vi "Menu Response.vi"(8 "error in (no error)":errorcluster, 10 "Menu Tag":string, 11 "Main in":refnum<class "Main.lvclass">) -> (0 "error out":errorcluster, 3 "Main out":refnum<class "Main.lvclass">)   [LabVIEW 2023, in "Main.lvlib" / "Main.lvclass"]
uses:
  Library/Main.lvclass
  Main Messages/Toggle Component Display Msg/Toggle Component Display Msg.lvclass/Toggle Component Display Msg.ctl
  builds/Framework/Engine.lvlibp/Engine/Accessors/Read Self Q.vi
  Custom Controls/Components.vi
  builds/Framework/Actor Framework.lvlibp/1abvi3w/vi.lib/ActorFramework/Message Enqueuer/Enqueue.vi
  builds/Framework/Actor Framework.lvlibp/1abvi3w/vi.lib/ActorFramework/Message Enqueuer/Message Enqueuer.lvclass
  <vilib>/ErrorRing/Error Ring.xnode
  Main Messages/Toggle Component Display Msg/Toggle Component Display Msg.lvclass
  Library/Main.lvclass/Main.ctl
  builds/Framework/Engine.lvlibp/Engine/Library/Engine.lvclass
  builds/Framework/Actor Framework.lvlibp/1abvi3w/vi.lib/ActorFramework/Stop Msg/Stop Msg.lvclass
  C:/Users/Public/Documents/Development/builds/Framework/Engine.lvlibp/Managed Actor/Library/Managed Actor.lvclass
  C:/Users/Public/Documents/Development/builds/Framework/Engine.lvlibp/Engine/Library/Engine.lvclass
  C:/Users/Public/Documents/Development/builds/Framework/Panel Manager.lvlibp/Library/Panel Actor.lvclass
  C:/Users/Public/Documents/Development/builds/Framework/Monitored Actor.lvlibp/Actor Monitor/Actor Monitor/Actor Monitor.lvclass
  C:/Users/Public/Documents/Development/builds/Framework/Actor Framework.lvlibp/1abvi3w/vi.lib/ActorFramework/Actor/Actor.lvclass
  C:/Users/Public/Documents/Development/Application/Main/Library/Main.lvclass
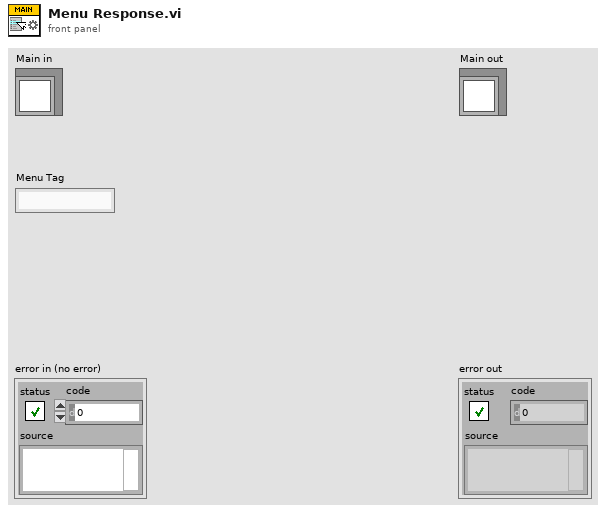
[diagram p1: front panel]
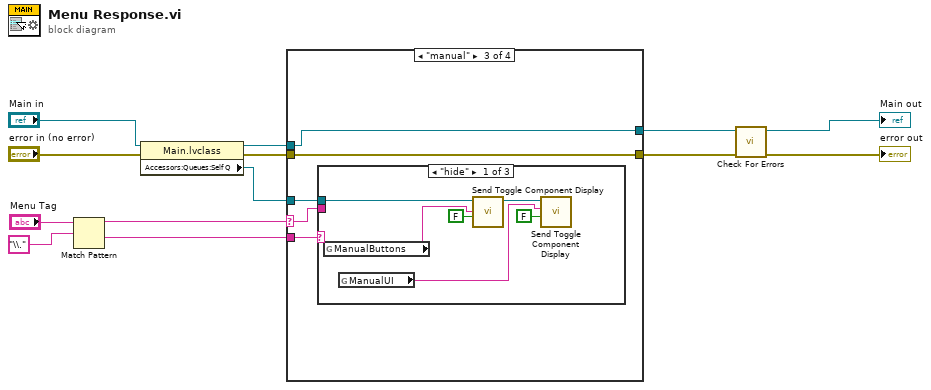
[diagram p0: block diagram]
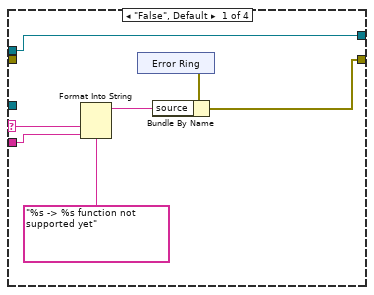
[diagram p2: hidden frame]
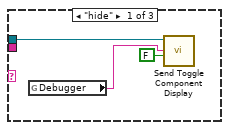
[diagram p4: hidden frame]
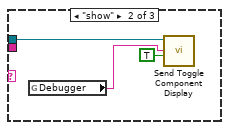
[diagram p5: hidden frame]
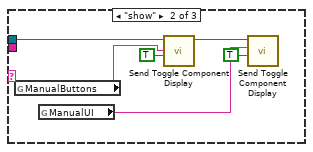
[diagram p6: hidden frame]
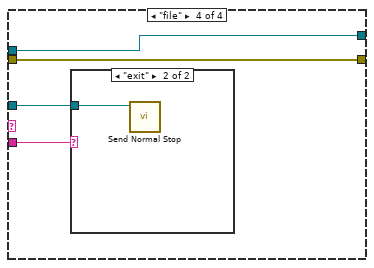
[diagram p8: hidden frame]
diagram:
  n1 = Match Pattern(string="Menu Tag", regular expression="\\.") -> (before substring=w10:string, after substring=w1:string)  [unwired: 1 in, 2 out]
  n2 = property class="Main.lvclass"(reference="Main in", error in="error in (no error)") -> (reference out=w9:refnum<class "Main.lvclass">, error out=w8:errorcluster, "Accessors:Queues:Self Q"=w2:refnum<class "Message Enqueuer.lvclass">)
  n3 = case shown="\"manual\"" w10 {
    selector: w10 -> [w15 w22 w33 _]
    tunnel: w9 -> [w20 w24 w35 w53]
    tunnel: w8 -> [_ w23 w34 w52]
    tunnel: [w20 w24 w35 w53] -> w5
    tunnel: [w16 w23 w34 w52] -> w4
    tunnel: w2 -> [_ w25 w36 w50]
    tunnel: w1 -> [w14 w26 w37 w51]
    frame "False", Default {
      n4 = Format Into String(format string="%s -> %s function not supported yet", w15, w14) -> (resulting string=w17:string)  [unwired: 2 in, 1 out]
      n5 = xnode "Error Ring"() -> ("error out"=w19:errorcluster)
      n6 = Bundle By Name(cluster=w19, "source"=w17) -> (w16:errorcluster)
    }
    frame "debugger" {
      n7 = case shown="Default" w26 {
        tunnel: w25 -> [w29 w32 _]
        tunnel: w22 -> [_ _ _]
        frame "hide" {
          n8 = global read "Components.vi" "Debugger"() -> (w27:string)
          n9 = call "Send Toggle Component Display.vi"("Show"=FALSE, "Identifier"=w27, "Message Enqueuer"=w29) -> ()  [unwired: 7 in, 2 out]
        }
        frame "show" {
          n10 = global read "Components.vi" "Debugger"() -> (w30:string)
          n11 = call "Send Toggle Component Display.vi"("Show"=TRUE, "Identifier"=w30, "Message Enqueuer"=w32) -> ()  [unwired: 7 in, 2 out]
        }
        frame Default {
        }
      }
    }
    frame "manual" {
      n12 = case shown="\"hide\"" w37 {
        tunnel: w36 -> [w43 w49 _]
        tunnel: w33 -> [_ _ _]
        frame "hide" {
          n13 = global read "Components.vi" "ManualButtons"() -> (w41:string)
          n14 = global read "Components.vi" "ManualUI"() -> (w38:string)
          n15 = call "Send Toggle Component Display.vi"("Show"=FALSE, "Identifier"=w41, "Message Enqueuer"=w43) -> ("Message Enqueuer out"=w39:refnum<class "Message Enqueuer.lvclass">)  [unwired: 7 in, 1 out]
          n16 = call "Send Toggle Component Display.vi"("Show"=FALSE, "Identifier"=w38, "Message Enqueuer"=w39) -> ()  [unwired: 7 in, 2 out]
        }
        frame "show" {
          n17 = global read "Components.vi" "ManualButtons"() -> (w47:string)
          n18 = global read "Components.vi" "ManualUI"() -> (w45:string)
          n19 = call "Send Toggle Component Display.vi"("Show"=TRUE, "Identifier"=w47, "Message Enqueuer"=w49) -> ("Message Enqueuer out"=w46:refnum<class "Message Enqueuer.lvclass">)  [unwired: 7 in, 1 out]
          n20 = call "Send Toggle Component Display.vi"("Show"=TRUE, "Identifier"=w45, "Message Enqueuer"=w46) -> ()  [unwired: 7 in, 2 out]
        }
        frame Default {
        }
      }
    }
    frame "file" {
      n21 = case shown="\"exit\"" w51 {
        tunnel: w50 -> [_ w54]
        frame "False", Default {
        }
        frame "exit" {
          n22 = call "Send Normal Stop.vi"("Message Enqueuer"=w54) -> ()  [unwired: 10 in, 1 out]
        }
      }
    }
  }
  n23 = call "Check For Errors.vi"("error in"=w4, "Engine in"=w5) -> ("error out"=→"error out":errorcluster, "Engine out"=→"Main out":refnum<class "Main.lvclass">)  [unwired: 8 in]
